vi "Get Client URI.vi"(11 "Processing in":refnum<class "Processing.lvclass">) -> (2 "Client URI":refnum<class "URI.lvclass">, 3 "Processing out":refnum<class "Processing.lvclass">)   [LabVIEW 2020, in "HTTP Server.lvlib" / "Processing.lvclass"]
uses:
  Processing.lvclass
  Processing.lvclass/Processing.ctl
  lv-uri/URI/URI/URI.lvclass
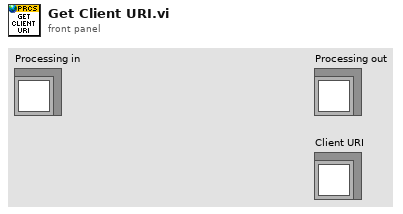
[diagram p1: front panel]
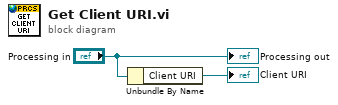
[diagram p0: block diagram]
diagram:
  n1 = Unbundle By Name("Processing in") -> ("Client URI"=→"Client URI":refnum<class "URI.lvclass">)
  "Processing out" <- "Processing in"
